vi "Archive Convergence Status.vi"(8 "error in":errorcluster, 10 "LBCB Filter":T1, 11 "Convergence Status":T2) -> (0 "error out":errorcluster, 2 "string":string)   [LabVIEW 2009]
uses:
  Mixed Mode Convergence Status.ctl
  Data Access Objects/Metadata/LBCB Filter.ctl
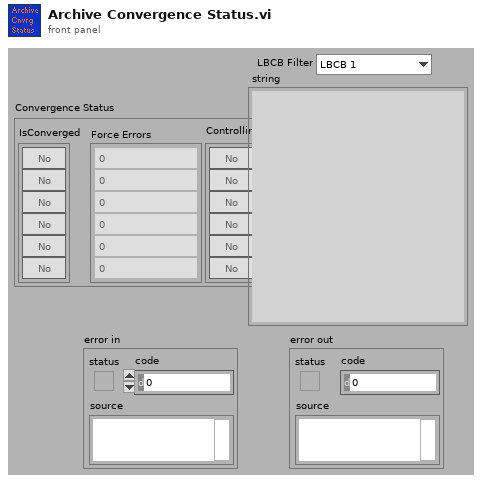
[diagram p1: front panel]
types:
  T1 = typedef "LBCB Filter.ctl" = enum16{"LBCB 1", "LBCB 2", "Both"}
  T2 = typedef "Mixed Mode Convergence Status.ctl" = cluster{"IsConverged":bool[], "Force Errors":dbl[], "Controlling DOF":bool[]}
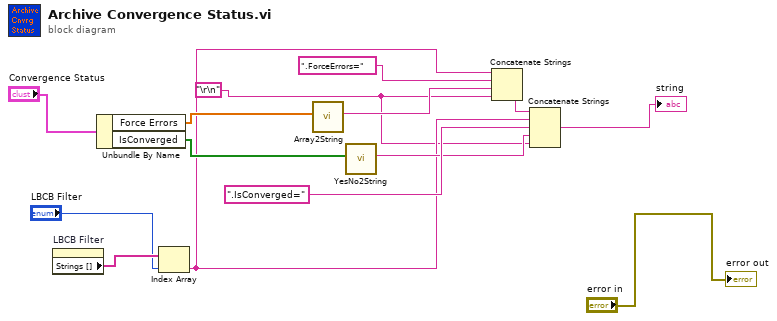
[diagram p0: block diagram]
diagram:
  w2 = "\r\n"
  n1 = property on="LBCB Filter" class="Enum (strict)"() -> ("Strings []"=w13:string[])  [unwired: 2 in, 2 out]
  n2 = Unbundle By Name("Convergence Status") -> ("Force Errors"=w10:dbl[], "IsConverged"=w6:bool[])
  n3 = Index Array(array=w13, index="LBCB Filter") -> (element=w4:string)
  n4 = call "Array2String.vi"("Array"=w10) -> ("String"=w9:string)  [unwired: 1 in, 9 out]
  n5 = call "YesNo2String.vi"("Yes/No"=w6) -> ("String"=w5:string)  [unwired: 10 out]
  n6 = Concatenate Strings(w4, ".ForceErrors=", w9, w2) -> (w8:string)
  n7 = Concatenate Strings(w8, w4, ".IsConverged=", w5, w2) -> (→"string":string)
  "error out" <- "error in"
